vi "GetMarks(SubVI).vi"(11 "connection reference 3":T1) -> (1 "Marks%":dbl, 2 "TotalMarks":string, 3 "connection reference 2":T1)   [LabVIEW 2013]
uses:
  <vilib>/addons/database/Connection.llb/Conn ObjectReference.ctl
  FYP_LabviewGlobal(SubVI).vi
  <vilib>/addons/database/_DB Variant To Data/Database Variant To Data.xnode
  <vilib>/addons/database/NI_Database_API.lvlib
panel:
  out "Numeric":dbl
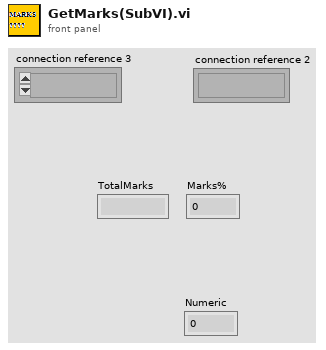
[diagram p1: front panel]
types:
  T1 = typedef "NI_Database_API.lvlib/Conn ObjectReference.ctl" = refnum<k1>
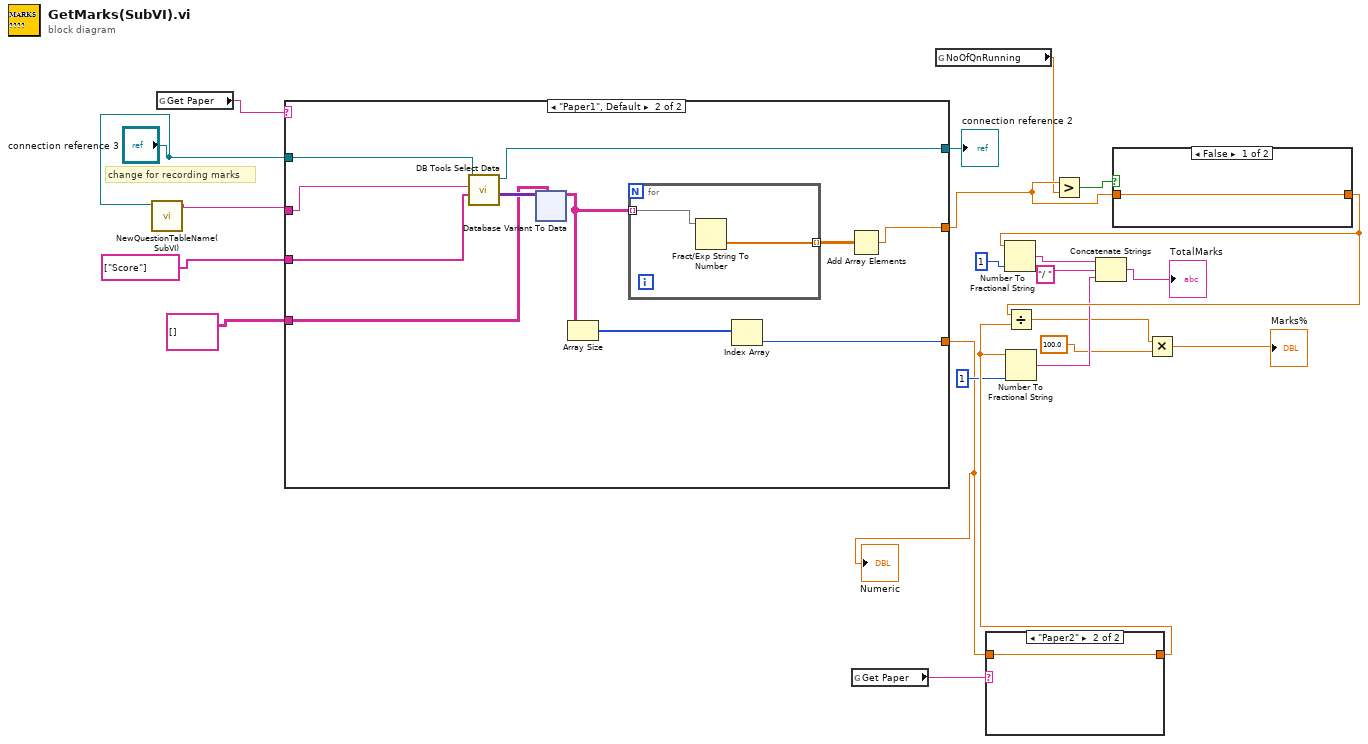
[diagram p0: block diagram]
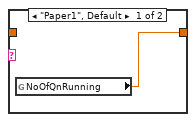
[diagram p2: hidden frame]
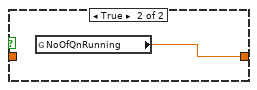
[diagram p3: hidden frame]
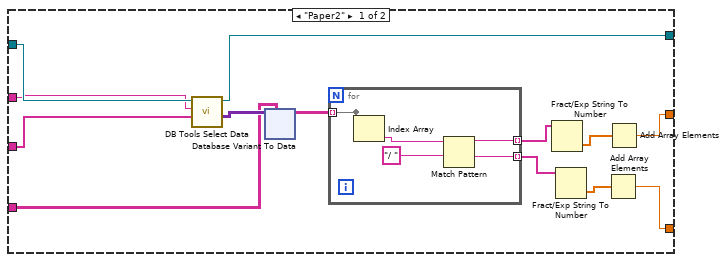
[diagram p4: hidden frame]
diagram:
  # "change for recording marks"
  n1 = call "NewQuestionTableName(SubVI).vi"("connection reference"="connection reference 3") -> ("String"=w2:string)  [unwired: 9 in, 1 out]
  n2 = global read "FYP_LabviewGlobal(SubVI).vi" "Get Paper"() -> (w22:string)
  n3 = case shown="\"Paper1\", Default" w22 {
    tunnel: w2 -> [w34 w94]
    tunnel: "connection reference 3" -> [w35 w95]
    tunnel: string[][] [] -> [w31 w92]
    tunnel: [w26 w89] -> w9
    tunnel: [w24 w88] -> w4
    tunnel: [w33 w86] -> w20
    tunnel: string[] ["Score"] -> [w23 w85]
    frame "Paper2" {
      n4 = call <vilib>:"DB Tools Select Data.vi"("columns"=w23, "table"=w34, "connection reference"=w35) -> ("data"=w32:variant[][], "connection reference out"=w33:T1)  [unwired: 3 in, 1 out]
      n5 = xnode "Database Variant To Data"("database variant"=w32, "type"=w31) -> ("data"=w30:string[][])  [unwired: 1 in, 1 out]
      n6 = for {
        tunnel: [w40] -> _ mode=indexing
        tunnel: w30 -> [w40] mode=indexing
        tunnel: [w37] -> w29 mode=indexing
        tunnel: [w36] -> w28 mode=indexing
        n7 = Index Array(array=w40) -> (element=w39:string)  [unwired: 1 in]
        n8 = Match Pattern(string=w39, regular expression="/ ") -> (before substring=w37:string, after substring=w36:string)  [unwired: 1 in, 2 out]
      }
      n9 = Fract/Exp String To Number(string=w29) -> (number=w27:dbl[])  [unwired: 3 in, 1 out]
      n10 = Fract/Exp String To Number(string=w28) -> (number=w25:dbl[])  [unwired: 3 in, 1 out]
      n11 = Add Array Elements(numeric array=w25) -> (sum=w24:dbl)
      n12 = Add Array Elements(numeric array=w27) -> (sum=w26:dbl)
    }
    frame "Paper1", Default {
      n13 = call <vilib>:"DB Tools Select Data.vi"("columns"=w85, "table"=w94, "connection reference"=w95) -> ("data"=w93:variant[][], "connection reference out"=w86:T1)  [unwired: 3 in, 1 out]
      n14 = xnode "Database Variant To Data"("database variant"=w93, "type"=w92) -> ("data"=w91:string[][])  [unwired: 1 in, 1 out]
      n15 = Array Size(array=w91) -> (size(s)=w87:i32[])
      n16 = for {
        tunnel: w91 -> [w97] mode=indexing
        tunnel: [w96] -> w90 mode=indexing
        n17 = Fract/Exp String To Number(string=w97) -> (number=w96:dbl[])  [unwired: 3 in, 1 out]
      }
      n18 = Index Array(array=w87) -> (element=w88:i32)  [unwired: 1 in]
      n19 = Add Array Elements(numeric array=w90) -> (sum=w89:dbl)
    }
  }
  "connection reference 2" <- w20
  "Numeric" <- w4
  n20 = global read "FYP_LabviewGlobal(SubVI).vi" "Get Paper"() -> (w6:string)
  n21 = global read "FYP_LabviewGlobal(SubVI).vi" "NoOfQnRunning"() -> (w7:dbl)
  n22 = case shown="\"Paper2\"" w6 {
    tunnel: w4 -> [_ w143]
    tunnel: [w142 w143] -> w12
    frame "Paper1", Default {
      n23 = global read "FYP_LabviewGlobal(SubVI).vi" "NoOfQnRunning"() -> (w142:dbl)
    }
    frame "Paper2" {
    }
  }
  n24 = Number To Fractional String(number=w12, precision (6)=i16 1) -> (F-format string=w14:string)  [unwired: 2 in]
  n25 = Greater?(x=w9, y=w7) -> (0:w19:bool)
  n26 = case shown="False" w19 {
    tunnel: [w144 w145] -> w15
    tunnel: w9 -> [w144 _]
    frame False {
    }
    frame True {
      n27 = global read "FYP_LabviewGlobal(SubVI).vi" "NoOfQnRunning"() -> (w145:dbl)
    }
  }
  n28 = Number To Fractional String(number=w15, precision (6)=i16 1) -> (F-format string=w17:string)  [unwired: 2 in]
  n29 = Divide(x=w15, y=w12) -> (x/y=w5:dbl)
  n30 = Concatenate Strings(w17, "/ " ("string"), w14) -> (→"TotalMarks":string)
  n31 = Multiply(x=w5, y=100.0) -> (x*y=→"Marks%":dbl)
